vi "IsPositionOccupied.vi"(10 "Position":T1, 11 "Board":bool[][](array[boolean])) -> (3 "Occupied?":bool)   [LabVIEW 2015, in "TronVIEWGameUtilities.lvlib"]
uses:
  TronVIEWGameUtilities.lvlib
  TronviewGame/Board/Position.ctl
  TronviewGame/Board/Board.lvclass
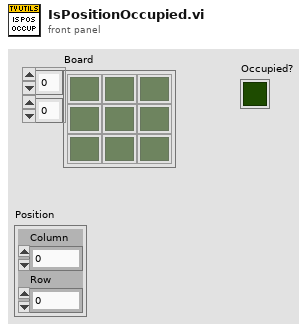
[diagram p1: front panel]
types:
  T1 = typedef "TronviewGame.lvlib/Board.lvclass/Position.ctl" = cluster{"Column":i32, "Row":i32}
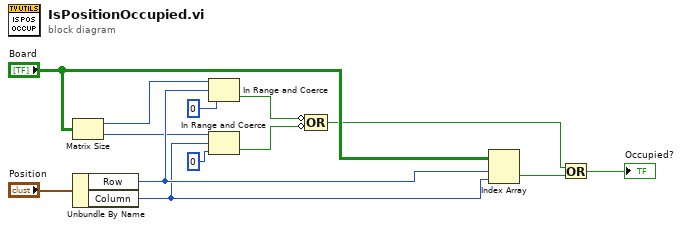
[diagram p0: block diagram]
diagram:
  n1 = Matrix Size(0:"Board") -> (1:w7:i32, 2:w3:i32)
  n2 = Unbundle By Name("Position") -> ("Row"=w8:i32, "Column"=w2:i32)
  n3 = In Range and Coerce(upper limit=w7, x=w8, lower limit=0) -> (In Range?=w6:bool)  [unwired: 1 out]
  n4 = In Range and Coerce(upper limit=w3, x=w2, lower limit=0) -> (In Range?=w1:bool)  [unwired: 1 out]
  n5 = Compound Arithmetic op=OR(invert w6, invert w1) -> (w10:bool)
  n6 = Index Array(array="Board", index (row)=w8, index (col)=w2) -> (element=w13:bool)
  n7 = Or(x=w10, y=w13) -> (x .or. y?=→"Occupied?":bool)
